vi "力特性 油压对应扭矩.vi"(7 "油压":dbl, 8 "油压B":dbl[](array[numeric]), 9 "油压A":dbl[](array[numeric]), 10 "扭矩B":dbl[](array[numeric]), 11 "扭矩A":dbl[](array[numeric])) -> (2 "油压扭矩左":dbl, 3 "油压扭矩右":dbl)   [LabVIEW 2015, in "Logging.lvlib"]
uses:
  Logging.lvlib
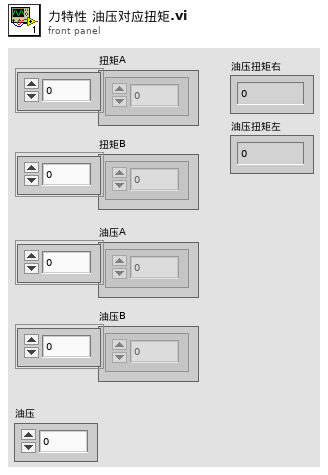
[diagram p1: front panel]
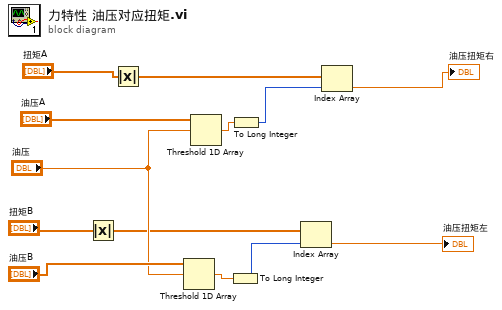
[diagram p0: block diagram]
diagram:
  n1 = Absolute Value(x="扭矩B") -> (abs(x)=w1:dbl[])
  n2 = Absolute Value(x="扭矩A") -> (abs(x)=w3:dbl[])
  n3 = Threshold 1D Array(2:"油压", 3:"油压B") -> (0:w13:dbl)  [unwired: 1 in]
  n4 = Threshold 1D Array(2:"油压", 3:"油压A") -> (0:w11:dbl)  [unwired: 1 in]
  n5 = To Long Integer(number=w13) -> (32bit integer=w12:i32)
  n6 = To Long Integer(number=w11) -> (32bit integer=w10:i32)
  n7 = Index Array(array=w1, index=w12) -> (element=→"油压扭矩左":dbl)
  n8 = Index Array(array=w3, index=w10) -> (element=→"油压扭矩右":dbl)
